vi "ReadTimeArray.vi"(8 "error in (no error)":errorcluster, 9 "dblTime Array":T1, 10 "ModuleID":i32) -> (0 "error out":errorcluster)   [LabVIEW 2017, in "EventModule.lvlib"]
uses:
  EventModule.lvlib
  PublicAPI/Arguments/Requests/dblTimeArray.ctl
  clEventType.ctl
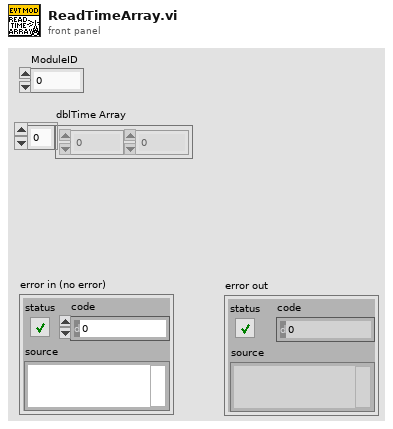
[diagram p1: front panel]
types:
  T1 = typedef "EventModule.lvlib/dblTimeArray.ctl" = dbl[]
  T2 = typedef "EventModule.lvlib/clEventType.ctl" = cluster{"ModuleID":i32, "Data":variant}
  T3 = typedef "EventModule.lvlib/clBroadcastEvents.ctl" = cluster{"DidInit":refnum<user-event>, "StatusUpdate":refnum<user-event>, "ErrorReport":refnum<user-event>, "DidStop":refnum<user-event>, "ReadEvtConfig":refnum<user-event>, "ReadTimeArray":refnum<user-event>, "ReadEvtParams":refnum<user-event>, "GetEvtReportArray":refnum<user-event>, "ReadPathToPlugin":refnum<user-event>, "GetEvtSignal":refnum<user-event>, "ReadBusNumber":refnum<user-event>}
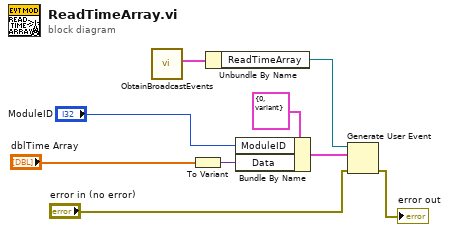
[diagram p0: block diagram]
diagram:
  n1 = call "ObtainBroadcastEvents.vi"() -> ("clBroadcastEvents"=w9:T3)  [unwired: 10 in, 1 out]
  n2 = To Variant(anything="dblTime Array") -> (Variant=w6:variant)
  n3 = Unbundle By Name(w9) -> ("ReadTimeArray"=w8:refnum<user-event>)
  n4 = Bundle By Name(cluster=T2 {"ModuleID"=0, "Data"=variant} ("clBroadcast"), "ModuleID"="ModuleID", "Data"=w6) -> (w5:T2)
  n5 = Generate User Event(user event=w8, event data cluster=w5, error in="error in (no error)") -> (error out=→"error out":errorcluster)  [unwired: 1 in, 1 out]
